vi "IMAQ DLL - Example.vi"() -> ()   [LabVIEW 2016]
panel:
  out "Row Column Indices":i32[][](array[numeric])
  out "Non Zero Px Total":u16
  in  "Array":u16[][](array[numeric])
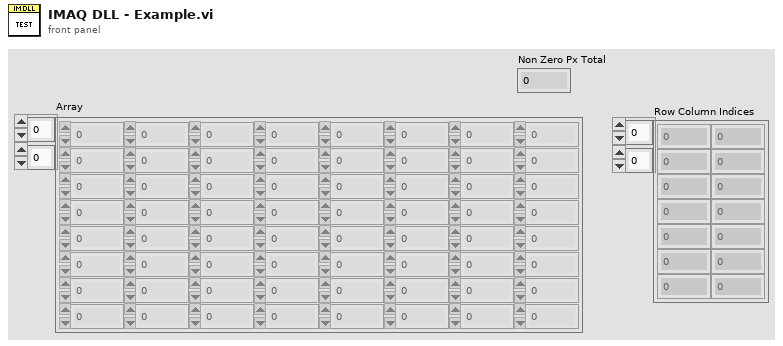
[diagram p1: front panel]
types:
  T1 = typedef "Image Type" = u32
  T2 = typedef "IMAQ Image.ctl" = refnum<image>
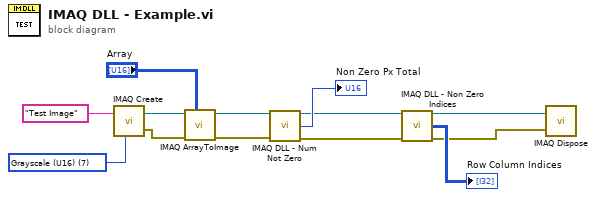
[diagram p0: block diagram]
diagram:
  w13 = T1 7 items=["Grayscale (U8)", "Grayscale (I16)", "Grayscale (SGL)", "Complex (CSG)", "RGB (U32)", "HSL (U32)", "RGB (U64)", "Grayscale (U16)"] ("Image Type")
  n1 = call "IMAQ Create"("Image Name"="Test Image", "Image Type"=w13) -> ("New Image"=w11:T2, "error out"=w8:errorcluster)  [unwired: 3 in]
  n2 = call "IMAQ ArrayToImage"("Image Pixels (U16)"="Array", "error in (no error)"=w8, "Image"=w11) -> ("error out"=w7:errorcluster, "Image Out"=w9:T2)  [unwired: 7 in]
  n3 = call "IMAQ DLL - Num Not Zero.vi"("IMAQ Ref"=w9, "Error In"=w7) -> ("IMAQ Ref (Dup)"=w5:T2, "Non Zero Px Total"=→"Non Zero Px Total":u16, "Error Out"=w4:errorcluster)  [unwired: 11 in]
  n4 = call "IMAQ DLL - Non Zero Indices.vi"("IMAQ Ref"=w5, "Error In"=w4) -> ("IMAQ Ref (Dup)"=w2:T2, "Row Column Indices"=→"Row Column Indices":i32[][], "Error Out"=w1:errorcluster)  [unwired: 10 in, 1 out]
  n5 = call "IMAQ Dispose"("Image"=w2, "error in (no error)"=w1) -> ()  [unwired: 4 in, 1 out]
